vi "Create.vi"(8 "error in (no error)":errorcluster, 9 "Index":i32, 10 "Card":string) -> (0 "error out":errorcluster, 3 "Card":refnum<class "Card.lvclass">)   [LabVIEW 2020, in "Card.lvclass"]
uses:
  Card.lvclass
  Card.lvclass/Card.ctl
panel:
  out "string array 2":string[](array[string])
  out "string array":string[](array[string])
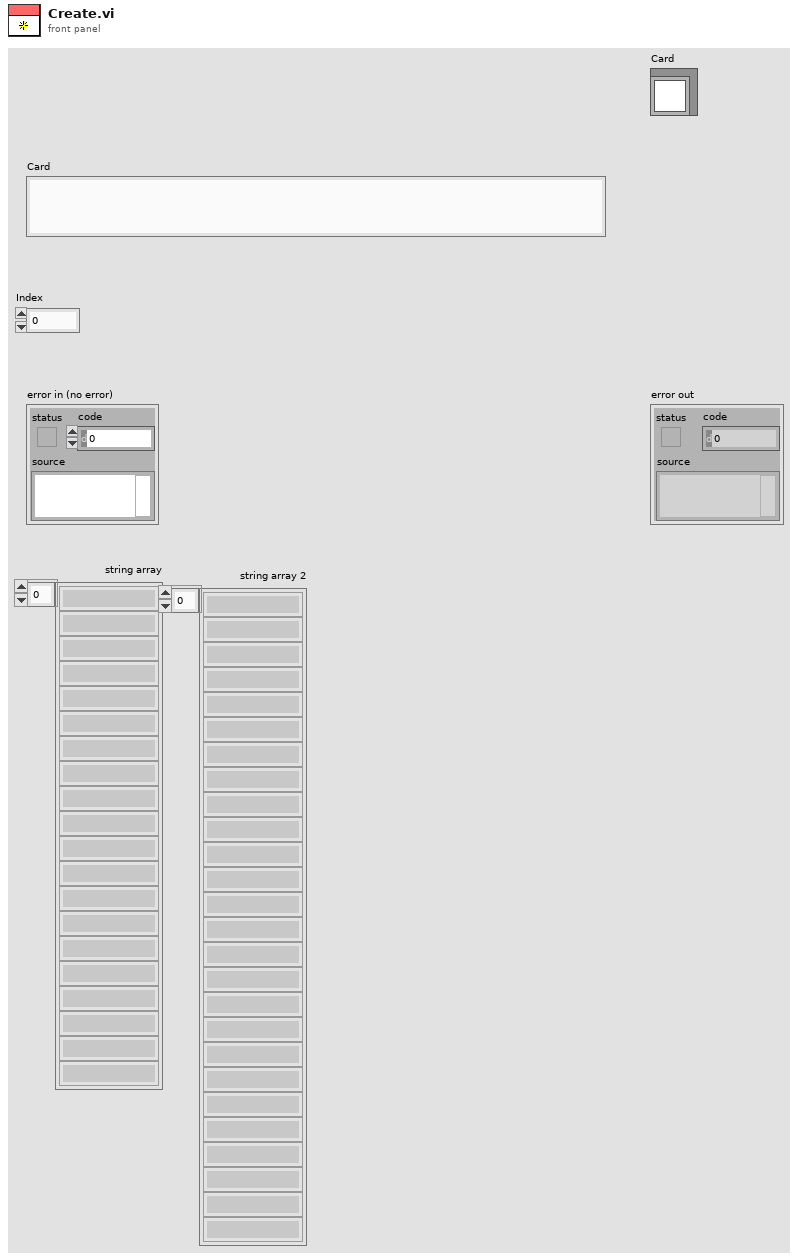
[diagram p1: front panel]
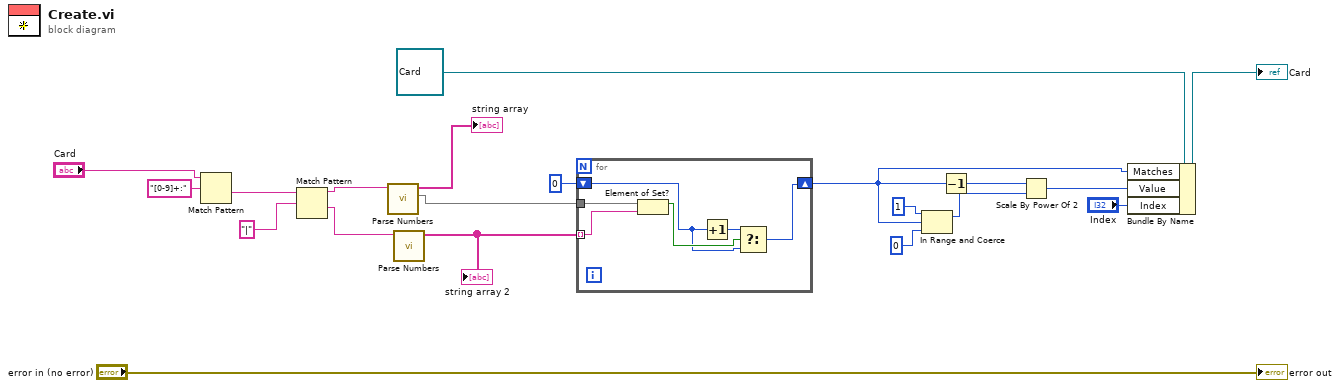
[diagram p0: block diagram]
diagram:
  n1 = Match Pattern(string="Card", regular expression="[0-9]+:") -> (after substring=w16:string)  [unwired: 1 in, 3 out]
  n2 = Match Pattern(string=w16, regular expression="|") -> (before substring=w14:string, after substring=w13:string)  [unwired: 1 in, 2 out]
  n3 = call "Parse Numbers.vi"("Card"=w14) -> ("set"=w12:set{string}, "string array"=→"string array":string[])  [unwired: 9 in]
  n4 = call "Parse Numbers.vi"("Card"=w13) -> ("string array"=w11:string[])  [unwired: 9 in, 1 out]
  "string array 2" <- w11
  n5 = for {
    tunnel: w12 -> [w26]
    tunnel: w11 -> [w25] mode=indexing
    shift-right: [w23] -> w2
    shift-left: 0 -> [w21]
    n6 = Element of Set?(10:w25, 11:w26) -> (3:w22:bool)
    n7 = Increment(x=w21) -> (x+1=w24:i32)
    n8 = Select(t=w24, s=w22, f=w21) -> (s? t:f=w23:i32)
  }
  n9 = In Range and Coerce(upper limit=1, x=w2, lower limit=0) -> (coerced(x)=w5:i32)  [unwired: 1 out]
  n10 = Decrement(x=w2) -> (x-1=w4:i32)
  n11 = Scale By Power Of 2(n=w4, x=w5) -> (x*2^n=w8:i32)
  n12 = Bundle By Name(cluster=refnum<class "Card.lvclass"> refnum ("Card"), "Matches"=w2, "Value"=w8, "Index"="Index") -> (→"Card":refnum<class "Card.lvclass">)
  "error out" <- "error in (no error)"
